vi "camera acquisition setup.vi"(0 "Camera Parameters (important)":T3={"Exposure Time (sec)"=0.1, "EM CCD Gain"=230, "Readout Settings"={"Acquisition Mode"=enum."Single Scan", "Pixel Rate"=enum."EM CCD 1 Mhz 16 bits", "High Capacity?"=FALSE, "V Shift Speed (us/row)"=enum."1.0  (not reccommended)", "V Shift Amplitude"=enum."+1", "Preamp Gain"=enum."2.6", "Trigger Mode"=0}, "Image Size"={"H Bin"=1, "V Bin"=1, "Left"=1, "Top"=1, "Right"=512, "Bottom"=512}, "Shutter"=0} {"Shutter" items=["Auto", "Stay Open", "Always Closed"]; "Readout Settings"."Trigger Mode" items=["Internal", "External"]; "EM CCD Gain" scale=0.01..255.0; "Exposure Time (sec)" scale=0.001..10.0 scale format="%#_1g"}) -> (14 "Image Size Out":T6={"H Bin"=1, "V Bin"=1, "Left"=1, "Top"=1, "Right"=512, "Bottom"=512} {"Top" min=4 max=2048 step=4; "Left" min=4 max=2048 step=4; "V Bin" min=1 max=2048 step=4; "H Bin" min=1 max=2048 step=4}, 15 "Continue with acq?":bool, 16 "File properties":T2 {"Max Space Req'd. (Gb)" format="%.2f"}, 19 "Error Out (no error)":errorcluster)   [LabVIEW 2014]
doc: "This VI sets the hardware and Glimpse parameters for acquisition from the Cascade camera. If requested, shows a live video preview to allow setting of acquisition AOI and other camera parameters. When user presses \"GO\", vi exits leaving camera setup. Intended for use as a sub-vi, interactively or non-.\n\nLimitations: does not display current temperatures"
uses:
  HAL Camera/image size - SubVI.ctl
  HAL Camera/HAL camera parameters important 1 - SubVI.ctl
  HAL Camera/ixon readout settings - SubVI.ctl
  HAL Camera/andor acquisition mode.ctl
  HAL Camera/file parameters 1 - SubVI.ctl
  <vilib>/vision/Image Controls.llb/IMAQ Image.ctl
  HAL Camera/camera globals - SubVI.vi
panel:
  in  "Laser Shutter":T1(radio)
  in  "Set to AOI":bool
  in  "Set to 512 x 300":bool
  in  "Set to Maximum":bool
  out "Actual Exposure Time (sec)":sgl format="%.4f"
  in  "Number of preview windows":i32=1
  in  "Go? (F)":bool
  in  "Quit":bool
  in  "Preview?":bool
  # "Information:"
  # "Parameters for non-interactive use"
  # "Camera: Andor iXon"
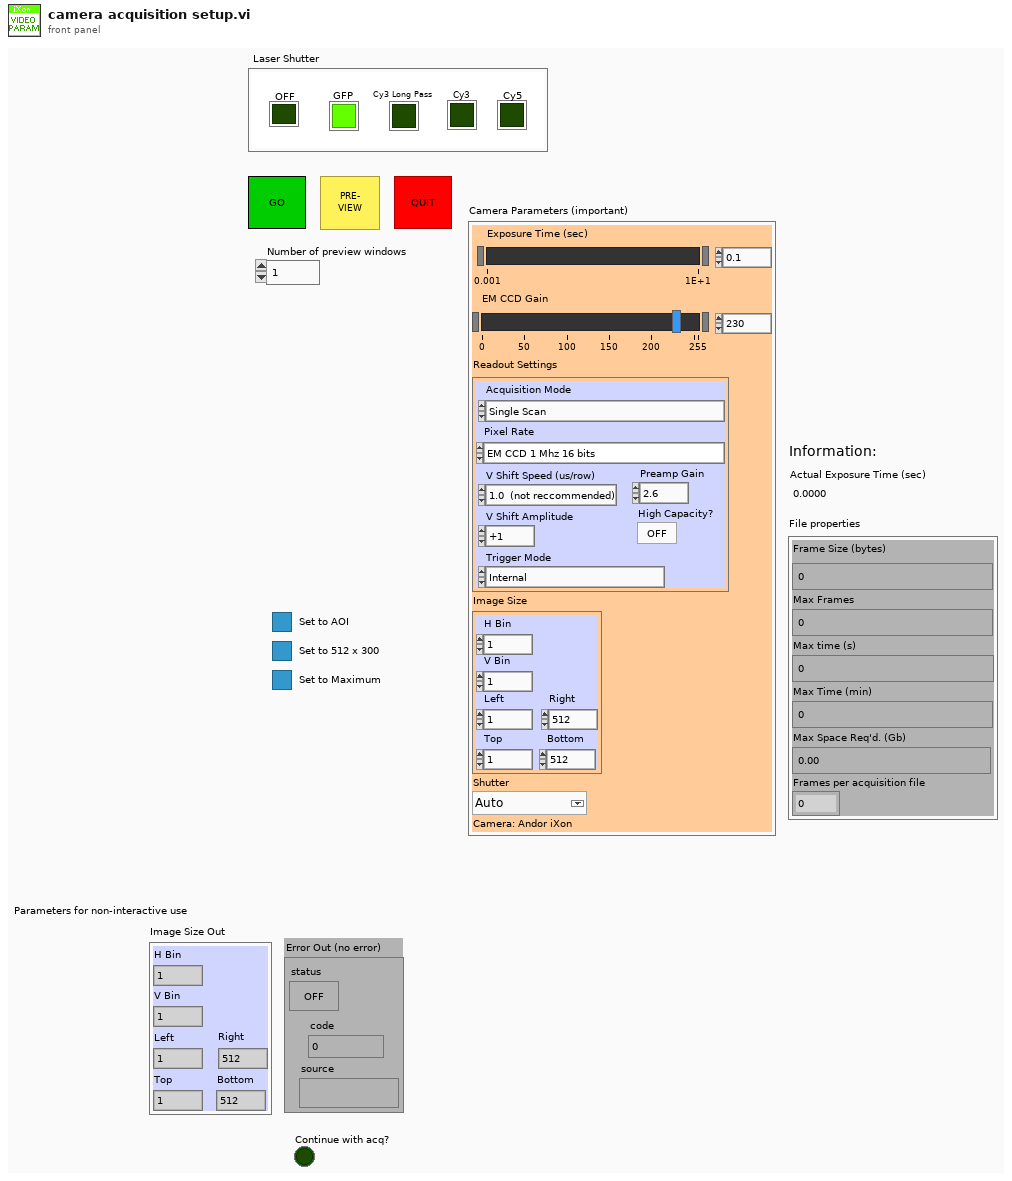
[diagram p1: front panel]
types:
  T1 = enum32{"GFP", "Cy3 Long Pass", "Cy3", "Cy5", "OFF"}
  T2 = typedef "file parameters 1 - SubVI.ctl" = cluster{"Frame Size (bytes)":u32, "Max Frames":u32, "Max time (s)":u32, "Max Time (min)":u32, "Max Space Req'd. (Gb)":dbl, "Frames per acquisition file":u32}
  T3 = typedef "HAL camera parameters important 1 - SubVI.ctl" = cluster{"Exposure Time (sec)":sgl, "EM CCD Gain":u8, "Readout Settings":T4, "Image Size":T6, "Shutter":i32}
  T4 = typedef "ixon readout settings - SubVI.ctl" = cluster{"Acquisition Mode":T5, "Pixel Rate":enum16{"EM CCD 10 Mhz 14 bits", "EM CCD 5 Mhz 14 bits", "EM CCD 3 Mhz 14 bits", "EM CCD 1 Mhz 16 bits", "Standard CCD 3 Mhz 14 bits", "Standard CCD 1 Mhz 16 bits"}, "High Capacity?":bool, "V Shift Speed (us/row)":enum16{"0.4 (not reccommended)", "0.6  (not reccommended)", "1.0  (not reccommended)", "1.8  (not reccommended)", "3.4  (not reccommended)", "6.6", "13.0"}, "V Shift Amplitude":enum16{"normal", "+1", "+2", "+3", "+4"}, "Preamp Gain":enum16{"1.0", "2.6"}, "Trigger Mode":u32}
  T5 = typedef "andor acquisition mode.ctl" = enum16{"(do not use)", "Single Scan", "Accumulate", "Kinetics", "Fast Kinetics", "Kinetics Run till Abort", "Frame Transfer", "Frame Transfer Run till Abort", "(do not use) ", "Time Delayed Integration"}
  T6 = typedef "image size - SubVI.ctl" = cluster{"H Bin":i32, "V Bin":i32, "Left":i32, "Top":i32, "Right":i32, "Bottom":i32}
  T7 = typedef "IMAQ Image.ctl" = refnum<image>
  T8 = typedef "ROI Descriptor" = cluster{"Global Rectangle":i32[], "Contours":cluster{"ID":enum32{"External", "Internal"}, "Type":u32, "Coordinates":i32[]}[]}
  T9 = typedef "andor camera properties - SubVI.ctl" = cluster{"Head Model":string, "Number of H pixels":i32, "Number of V pixels":i32, "Minimum temperature":i32, "Maximum temperature":i32}
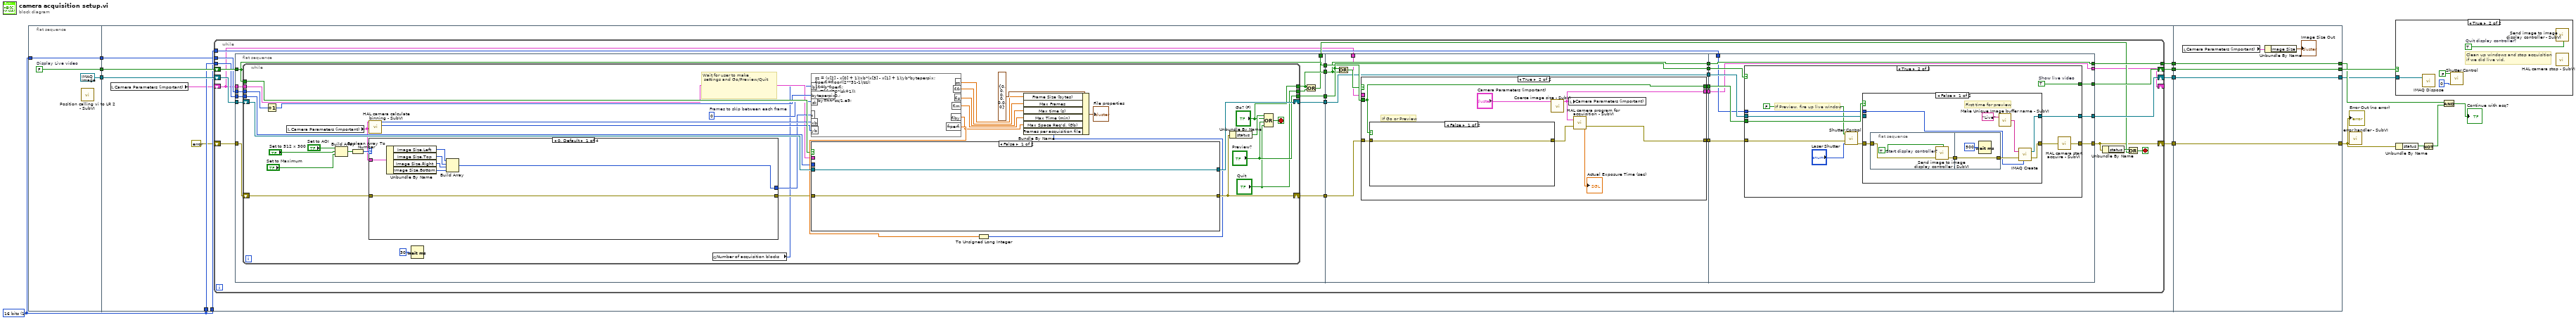
[diagram p0: block diagram]
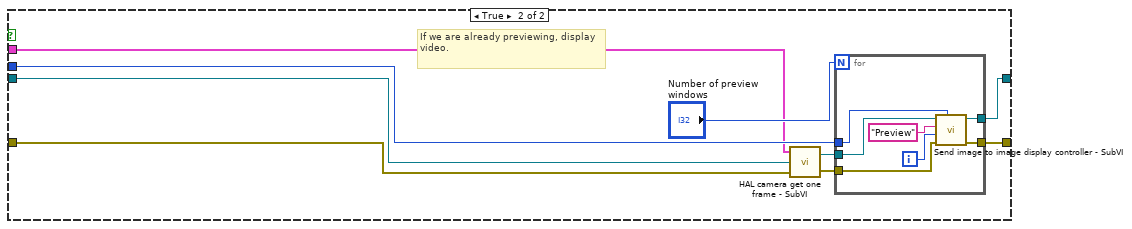
[diagram p2: hidden frame]
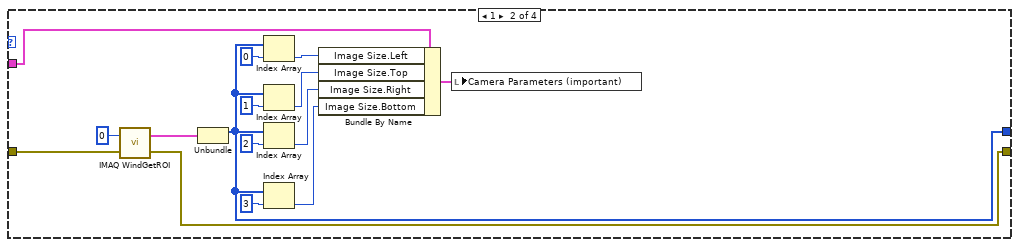
[diagram p3: hidden frame]
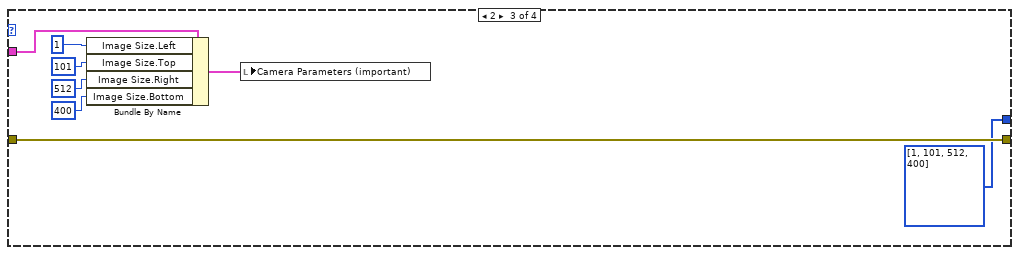
[diagram p4: hidden frame]
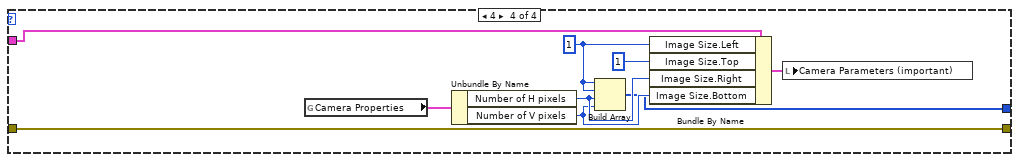
[diagram p5: hidden frame]
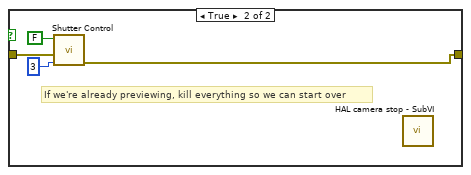
[diagram p7: hidden frame]
diagram:
  w8 = u32 1 items=["8 bits", "16 bits", "Float", "Complex", "RGB", "HSL"] ("Image Type")
  n1 = flat-sequence {
    tunnel: [w18] -> w13
    tunnel: [T7 refnum ("New Image")] -> w11
    tunnel: w8 -> [w16]
    tunnel: [w16] -> w7
    tunnel: w13 -> [w29]
    tunnel: w11 -> [w25]
    tunnel: w8 -> [w23]
    tunnel: w8 -> [w22]
    tunnel: w7 -> [w21]
    tunnel: [w28] -> w6
    tunnel: [w27] -> w5
    tunnel: [w26] -> w4
    tunnel: [w24] -> w3
    tunnel: [w227] -> w10
    tunnel: [w228] -> w14
    tunnel: [w229] -> w2
    tunnel: [w230] -> w15
    tunnel: w6 -> [w230]
    tunnel: w5 -> [w229]
    tunnel: w4 -> [w228]
    tunnel: w3 -> [w227]
    frame #0 {
      w18 = FALSE  # Display Live video
      n2 = call "Position calling vi to LR 2 - SubVI.vi"() -> ()  [unwired: 4 in, 2 out]
    }
    frame #1 {
      n3 = local read "Camera Parameters (important)"() -> (w19:T3)
      n4 = while {
        shift-right: [w53] -> w28
        shift-left: w29 -> [w55]
        shift-right: [w52] -> w24
        shift-left: w25 -> [w42]
        shift-right: [w33] -> w27
        shift-left: errorcluster {"status"=FALSE, "code"=0, "source"=""} ("error out") -> [w54]
        tunnel: [w51] -> w26
        tunnel: w23 -> [w36]
        tunnel: w22 -> [w35]
        tunnel: w21 -> [w34]
        shift-right: [w31] -> _
        shift-left: w19 -> [w30]
        stop <- w41 stop-if-true
        n5 = flat-sequence {
          tunnel: w55 -> [w67]
          tunnel: [w67] -> w50
          tunnel: w42 -> [w66]
          tunnel: w54 -> [w65]
          tunnel: [w64] -> w49
          tunnel: [w61] -> w48
          tunnel: [w63] -> w47
          tunnel: [w60] -> w39
          tunnel: [w59] -> w38
          tunnel: w36 -> [w58]
          tunnel: w34 -> [w57]
          tunnel: w30 -> [w56]
          tunnel: w50 -> [w167]
          tunnel: [w164] -> w46
          tunnel: [w170] -> w45
          tunnel: w49 -> [w169]
          tunnel: w48 -> [w164]
          tunnel: w47 -> [w168]
          tunnel: [w168] -> w44
          tunnel: [w165] -> w43
          tunnel: w38 -> [w163]
          tunnel: [w163] -> w37
          tunnel: [w162] -> w32
          tunnel: w30 -> [w161]
          tunnel: w43 -> [w193]
          tunnel: [w192] -> w53
          tunnel: [w191] -> w52
          tunnel: [w190] -> w33
          tunnel: [w189] -> w51
          tunnel: w46 -> [w189]
          tunnel: w45 -> [w194]
          tunnel: w44 -> [w195]
          tunnel: w37 -> [w188]
          tunnel: w35 -> [w187]
          tunnel: w32 -> [w186]
          tunnel: [w186] -> w31
          frame #0 {
            n6 = while {
              shift-left: w65 -> [w97]
              shift-right: [w92] -> w64
              tunnel: ["Go? (F)"] -> w61
              tunnel: w67 -> [w94]
              tunnel: ["Preview?"] -> w63
              tunnel: ["Quit"] -> w62
              shift-right: [w90] -> w59
              shift-left: w66 -> [w98]
              tunnel: w58 -> [w89]
              tunnel: w57 -> [w87]
              tunnel: w56 -> [w78]
              stop <- w79 stop-if-true
              w93 = u16 0  # Frames to skip between each frame
              # "Wait for user to make\n settings and Go/Preview/Quit"
              n7 = Increment(x=w87) -> (x+1=w88:u32)
              n8 = local read "Camera Parameters (important)"() -> (w77:T3)
              n9 = Build Array("Set to AOI", "Set to 512 x 300", "Set to Maximum") -> (w103:bool[])
              n10 = Boolean Array To Number(Boolean array=w103) -> (number=w99:u32)
              n11 = call "HAL camera calculate binning - SubVI.vi"("Camera Parameters (important)"=w77) -> ("V Bin"=w85:i32, "H Bin"=w86:i32)  [unwired: 9 in]
              n12 = case shown="0, Default" w99 {
                tunnel: w97 -> [w128 w143 w151 w160]
                tunnel: [w122 w136 i32[] [1, 101, 512, 400] ("Global Rectangle") w152] -> w84
                tunnel: [w128 w141 w151 w160] -> w91
                tunnel: w77 -> [w123 w129 w144 w157]
                frame 0, Default {
                  n13 = Unbundle By Name(w123) -> ("Image Size.Left"=w124:i32, "Image Size.Top"=w125:i32, "Image Size.Right"=w126:i32, "Image Size.Bottom"=w127:i32)
                  n14 = Build Array(w124, w125, w126, w127) -> (w122:i32[])
                }
                frame 1 {
                  n15 = call "IMAQ WindGetROI"("Window Number (0...15)"=0, "error in (no error)"=w143) -> ("ROI Descriptor"=w142:T8, "error out"=w141:errorcluster)  [unwired: 3 out]
                  n16 = Unbundle(w142) -> ("Global Rectangle"=w136:i32[])  [unwired: 1 out]
                  n17 = Index Array(array=w136, index=0) -> (element=w134:i32)
                  n18 = Index Array(array=w136, index=1) -> (element=w133:i32)
                  n19 = Index Array(array=w136, index=2) -> (element=w132:i32)
                  n20 = Index Array(array=w136, index=3) -> (element=w131:i32)
                  n21 = Bundle By Name(cluster=w129, "Image Size.Left"=w134, "Image Size.Top"=w133, "Image Size.Right"=w132, "Image Size.Bottom"=w131) -> (w135:T3)
                  n22 = local write "Camera Parameters (important)"(w135) -> ()
                }
                frame 2 {
                  n23 = Bundle By Name(cluster=w144, "Image Size.Left"=1 ("Left"), "Image Size.Top"=101 ("Top"), "Image Size.Right"=512 ("Right"), "Image Size.Bottom"=400 ("Bottom")) -> (w148:T3)
                  n24 = local write "Camera Parameters (important)"(w148) -> ()
                }
                frame 4 {
                  w155 = 1 ("Left")
                  n25 = global read "camera globals - SubVI.vi" "Camera Properties"() -> (w156:T9)
                  n26 = Unbundle By Name(w156) -> ("Number of H pixels"=w154:i32, "Number of V pixels"=w153:i32)
                  n27 = Build Array(w155, w155, w154, w153) -> (w152:i32[])
                  n28 = Bundle By Name(cluster=w157, "Image Size.Left"=w155, "Image Size.Top"=1 ("Top"), "Image Size.Right"=w154, "Image Size.Bottom"=w153) -> (w159:T3)
                  n29 = local write "Camera Parameters (important)"(w159) -> ()
                }
              }
              n30 = Wait (ms)(milliseconds to wait=u32 30) -> ()  [unwired: 1 out]
              n31 = global read "camera globals - SubVI.vi" "Number of acquisition blocks"() -> (w76:i8)
              n32 = formula code="sz = (x[2] - x[0] + 1)/xb*(x[3] - x[1] + 1)/yb*byteperpix;\nfrperfi=floor((2**31-1)/sz);\nfifr=b*frperfi;\nfis=fifr/(30*(sk+1));\nfim=fis/60.;\nfiby=fifr*sz/1.e9;"("x"=w84, "b"=w76, "sk"=w93, "xb"=w86, "yb"=w85, "byteperpix"=w88) -> ("sz"=w69:dbl, "fifr"=w68:dbl, "fis"=w70:dbl, "fim"=w71:dbl, "fiby"=w72:dbl, "frperfi"=w95:dbl)
              n33 = case shown="False" w94 {
                tunnel: w98 -> [w104 w113]
                tunnel: [w105 w111] -> w92
                tunnel: w91 -> [w105 w114]
                tunnel: [w104 w112] -> w90
                tunnel: w89 -> [_ w107]
                tunnel: w78 -> [_ w106]
                frame False {
                }
                frame True {
                  # "If we are already previewing, display video."
                  n34 = call "HAL camera get one frame - SubVI.vi"("error in"=w114, "New Image"=w113, "Camera Parameters (important)"=w106) -> ("error out"=w110:errorcluster, "Image Out"=w108:T7)
                  n35 = for {
                    N: "Number of preview windows" -> [_]
                    tunnel: [w121] -> w112
                    tunnel: [w120] -> w111
                    tunnel: w110 -> [w119]
                    tunnel: w108 -> [w118]
                    tunnel: w107 -> [w115]
                    i -> [w116]
                    n36 = call "Send image to image display controller - SubVI.vi"("Image"=w118, "Window Title"="Preview" ("Window Title\n(Window only)"), "Window Number"=w116, "error in"=w119, "Image Type"=w115) -> ("Image Out"=w121:T7, "error out"=w120:errorcluster)  [unwired: 4 in]
                  }
                }
              }
              n37 = To Unsigned Long Integer(number=w95) -> (unsigned 32bit integer=w73:u32)
              n38 = Bundle By Name(cluster=T2 {"Frame Size (bytes)"=0, "Max Frames"=0, "Max time (s)"=0, "Max Time (min)"=0, "Max Space Req'd. (Gb)"=0.0, "Frames per acquisition file"=0} ("Glimpse file properties"), "Frame Size (bytes)"=w69, "Max Frames"=w68, "Max time (s)"=w70, "Max Time (min)"=w71, "Max Space Req'd. (Gb)"=w72, "Frames per acquisition file"=w73) -> (→"File properties":T2)
              n39 = Unbundle By Name(w92) -> ("status"=w83:bool)
              n40 = Compound Arithmetic op=OR(w83, "Go? (F)", "Preview?", "Quit") -> (w79:bool)
            }
            n41 = Or(x=w61, y=w62) -> (x .or. y?=w60:bool)
          }
          frame #1 {
            n42 = Or(x=w168, y=w164) -> (x .or. y?=w166:bool)
            n43 = case shown="True" w166 {
              tunnel: [w173 w176] -> w170
              tunnel: w169 -> [w173 w179]
              tunnel: w167 -> [w172 w180]
              tunnel: [w172 w180] -> w165
              tunnel: [w171 w174] -> w162
              tunnel: w161 -> [w171 _]
              frame False {
              }
              frame True {
                # "If Go or Preview"
                n44 = case shown="False" w180 {
                  tunnel: w179 -> [w181 w185]
                  tunnel: [w181 w184] -> w178
                  frame False {
                  }
                  frame True {
                    # "If we're already previewing, kill everything so we can start over"
                    n45 = call "Shutter Control.vi"("Laser Shutter"=3, "error in"=w185, "Camera Shutter"=FALSE) -> ("error out"=w184:errorcluster)  [unwired: 8 in]
                    n46 = call "HAL camera stop - SubVI.vi"() -> ()  [unwired: 1 in]
                  }
                }
                n47 = call "Coerce image size - SubVI.vi"("Camera Parameters (important) in"="Camera Parameters (important)") -> ("Camera Parameters (important) out"=w174:T3)  [unwired: 10 in]
                n48 = local write "Camera Parameters (important)"(w174) -> ()
                n49 = call "HAL camera program for acquisition - SubVI.vi"("error in"=w178, "Camera Parameters (important)"=w174) -> ("error out"=w176:errorcluster, "Actual Exposure Time (sec)"=→"Actual Exposure Time (sec)":sgl)
              }
            }
          }
          frame #2 {
            n50 = case shown="True" w195 {
              tunnel: w194 -> [w197 w203]
              tunnel: [w198 w209] -> w192
              tunnel: w193 -> [w198 w207]
              tunnel: [w196 w208] -> w191
              tunnel: [w197 w204] -> w190
              tunnel: w188 -> [w196 w206]
              tunnel: w187 -> [_ w205]
              frame False {
              }
              frame True {
                w209 = TRUE  # Show live video
                # "If Preview, fire up live window"
                n51 = call "Shutter Control.vi"("Laser Shutter"="Laser Shutter", "error in"=w203, "Camera Shutter"=FALSE) -> ("error out"=w202:errorcluster)  [unwired: 8 in]
                n52 = case shown="False" w207 {
                  tunnel: [w217 w223] -> w199
                  tunnel: [w214 w224] -> w208
                  tunnel: w206 -> [_ w224]
                  tunnel: w205 -> [w210 _]
                  tunnel: w202 -> [w213 w223]
                  frame False {
                    # "First time for preview"
                    n53 = flat-sequence {
                      tunnel: w213 -> [w219]
                      tunnel: [w218] -> w211
                      tunnel: [w222] -> w212
                      tunnel: w211 -> [w222]
                      frame #0 {
                        w220 = TRUE  # Start display controller?
                        n54 = call "Send image to image display controller - SubVI.vi"("error in"=w219, "Start display controller?"=w220) -> ("error out"=w218:errorcluster)  [unwired: 7 in, 1 out]
                      }
                      frame #1 {
                        n55 = Wait (ms)(milliseconds to wait=u32 500) -> ()  [unwired: 1 out]
                      }
                    }
                    n56 = call "Make Unique Image buffer name - SubVI.vi"("Buffer  base name"="Live" ("Image Name")) -> ("Image Name"=w215:string)  [unwired: 1 in]
                    n57 = call "IMAQ Create"("Image Name"=w215, "Image Type"=w210, "error in (no error)"=w212) -> ("New Image"=w214:T7, "error out"=w217:errorcluster)  [unwired: 1 in, 1 out]
                  }
                  frame True {
                  }
                }
                n58 = call "HAL camera start acquire - SubVI.vi"("error in"=w199) -> ("error out"=w204:errorcluster)
              }
            }
          }
        }
        n59 = Unbundle By Name(w33) -> ("status"=w40:bool)
        n60 = Or(x=w40, y=w39) -> (x .or. y?=w41:bool)
      }
    }
    frame #2 {
      n61 = local read "Camera Parameters (important)"() -> (w226:T3)
      n62 = Unbundle By Name(w226) -> ("Image Size"=→"Image Size Out":T6)
    }
  }
  n63 = call "error handler - SubVI.vi"("error in"=w2) -> ()  [unwired: 4 in, 3 out]
  n64 = case shown="True" w15 {
    tunnel: w10 -> [_ w234]
    frame False {
    }
    frame True {
      w233 = TRUE  # Quit display controller?
      # "Clean up windows and stop acquisition\nif we did live vid."
      n65 = call "IMAQ Dispose"("Image"=w234) -> ()  [unwired: 2 in, 4 out]
      n66 = call "Shutter Control.vi"("Laser Shutter"=0, "Camera Shutter"=FALSE) -> ()  [unwired: 9 in, 1 out]
      n67 = call "Send image to image display controller - SubVI.vi"("Quit display controller?"=w233) -> ()  [unwired: 8 in, 2 out]
      n68 = call "HAL camera stop - SubVI.vi"() -> ()  [unwired: 1 in]
    }
  }
  n69 = Unbundle By Name(w2) -> ("status"=w9:bool)
  n70 = Not(x=w9) -> (.not. x?=w12:bool)
  n71 = And(x=w14, y=w12) -> (x .and. y?=→"Continue with acq?":bool)
  "Error Out (no error)" <- w2
